vi "SetVertical.vi"(7 "coupling":i32, 8 "Offset":dbl, 9 "Range":dbl, 10 "AnalogChannel":refnum<k24>, 11 "SmartScope in":refnum<k24>) -> (0 "GraphMin":dbl, 1 "GraphMax":dbl, 3 "SmartScope out":refnum<k24>, 4 "OffsetMax":dbl, 6 "OffsetMin":dbl)   [LabVIEW 2013]
uses:
  C:/Program Files (x86)/LabNation/SmartScope/DeviceInterface.dll
  Program Files (x86)/LabNation/SmartScope/DeviceInterface.dll
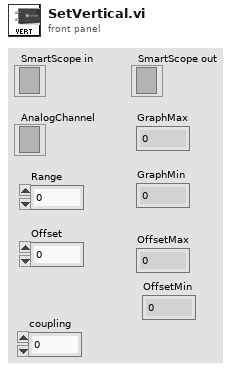
[diagram p1: front panel]
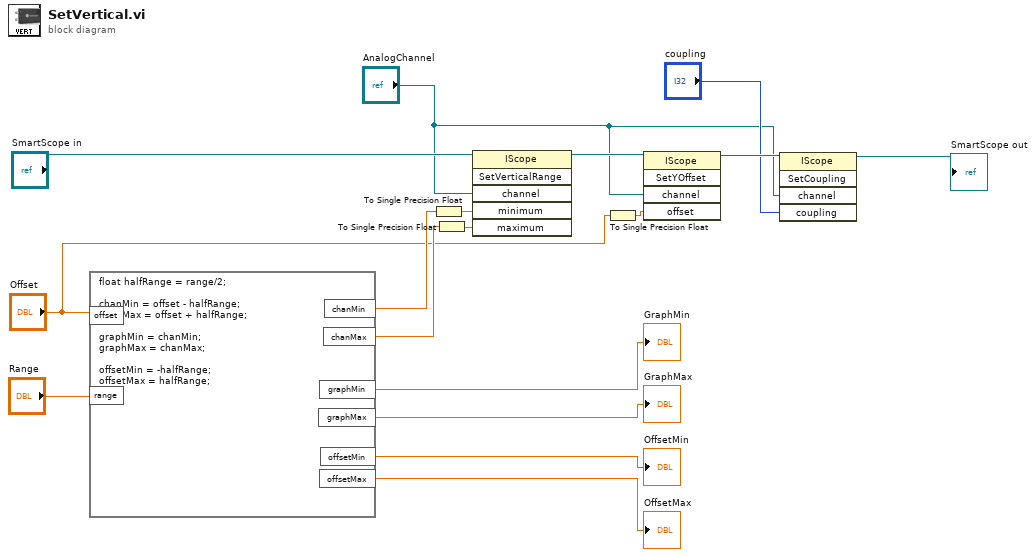
[diagram p0: block diagram]
diagram:
  n1 = formula code="float halfRange = range/2;\n\nchanMin = offset - halfRange;\nchanMax = offset + halfRange;\n\ngraphMin = chanMin;\ngraphMax = chanMax;\n\noffsetMin = -halfRange;\noffsetMax = halfRange;"("range"="Range", "offset"="Offset") -> ("chanMin"=w5:dbl, "chanMax"=w3:dbl, "offsetMin"=→"OffsetMin":dbl, "offsetMax"=→"OffsetMax":dbl, "graphMin"=→"GraphMin":dbl, "graphMax"=→"GraphMax":dbl)
  n2 = To Single Precision Float(number=w5) -> (single precision float=w6:sgl)
  n3 = To Single Precision Float(number=w3) -> (single precision float=w4:sgl)
  n4 = invoke class="IScope" method="SetVerticalRange"(reference="SmartScope in", "channel"="AnalogChannel", "minimum"=w6, "maximum"=w4) -> (reference out=w8:refnum<k24>)  [unwired: 2 in, 5 out]
  n5 = To Single Precision Float(number="Offset") -> (single precision float=w2:sgl)
  n6 = invoke class="IScope" method="SetYOffset"(reference=w8, "channel"="AnalogChannel", "offset"=w2) -> (reference out=w17:refnum<k24>)  [unwired: 2 in, 4 out]
  n7 = invoke class="IScope" method="SetCoupling"(reference=w17, "channel"="AnalogChannel", "coupling"="coupling") -> (reference out=→"SmartScope out":refnum<k24>)  [unwired: 2 in, 4 out]
